vi "fit_data.vi"() -> ()   [LabVIEW 2013]
uses:
  <vilib>/Analysis/6fits.llb/Curve Fitting Criteria.ctl
  <vilib>/Analysis/6fits.llb/Confidence Interval (Linear).vi
  <vilib>/Utility/file.llb/Read From Spreadsheet File (DBL).vi
  <vilib>/Analysis/NI_AALPro.lvlib
panel:
  out "RMSE 2":dbl
  out "R-square":dbl
  out "SSE":dbl
  in  "confidence level":dbl=0.67 format="%.2f"
  out "delta intercept":dbl
  out "RMSE":dbl
  out "residue":dbl format="%#_3g"
  out "intercept":dbl
  out "XY Graph":T1(graph)
  in  "data file":path=path "C:/Users/Thermo/Documents/GitHub/HelixMC/MSControl/test_vis/fit_data_linear.txt"
  in  "Combo Box":string(combo)
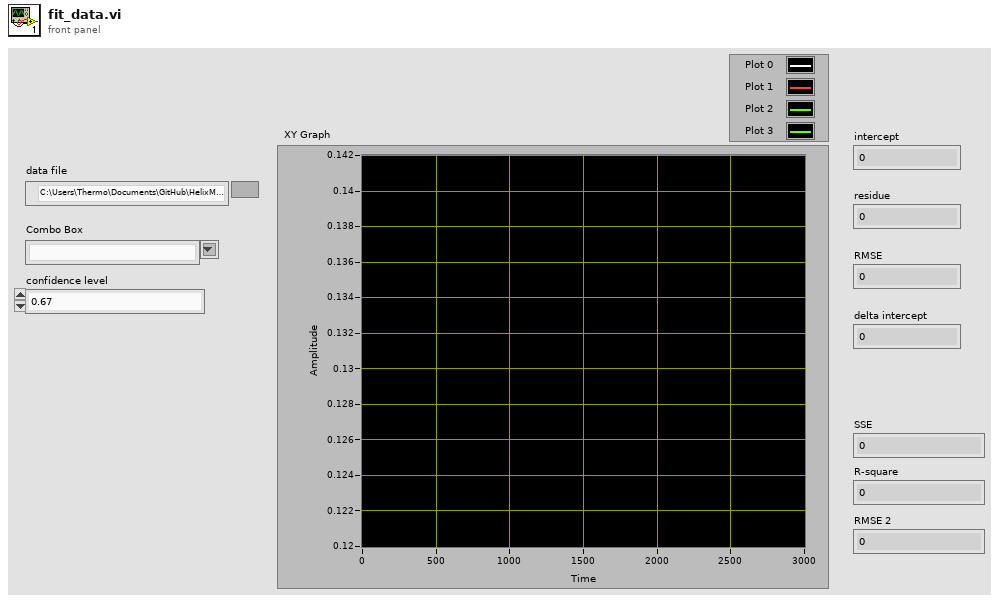
[diagram p1: front panel]
types:
  T1 = cluster{"all rows":dbl[], "Best Linear Fit":dbl[]}[]
  T2 = typedef "NI_AALPro.lvlib/Curve Fitting Criteria.ctl" = u16
  T3 = cluster{"all rows":dbl[], "Best Linear Fit":dbl[]}
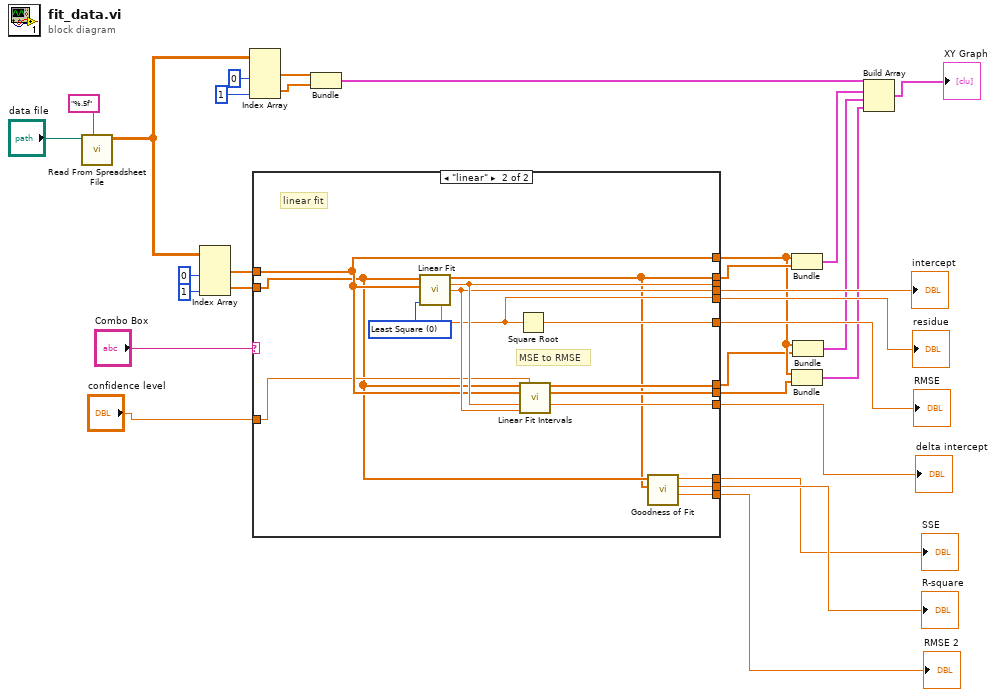
[diagram p0: block diagram]
diagram:
  n1 = call-poly <vilib>:"Read From Spreadsheet File.vi"("format (%.3f)"="%.5f", "file path (dialog if empty)"="data file") -> ("all rows"=w22:dbl[][])  [unwired: 5 in, 4 out]
  n2 = Index Array(array=w22, index (col) #1=0 ("disabled index (col)"), index (col) #2=1 ("index (col)")) -> (element #1=w24:dbl[], element #2=w23:dbl[])  [unwired: 2 in]
  n3 = Index Array(array=w22, index (col) #1=0 ("disabled index (col)"), index (col) #2=1 ("index (col)")) -> (element #1=w19:dbl[], element #2=w18:dbl[])  [unwired: 2 in]
  n4 = case shown="\"linear\"" "Combo Box" {
    tunnel: w24 -> [w30 w37]
    tunnel: w23 -> [_ w35]
    tunnel: [_ w34] -> w17
    tunnel: [_ w44] -> _
    tunnel: [_ w43] -> w13
    tunnel: [_ w42] -> w12
    tunnel: [_ w41] -> w11
    tunnel: [_ w40] -> w8
    tunnel: [_ w39] -> w7
    tunnel: [_ w38] -> w4
    tunnel: [w30 w37] -> w9
    tunnel: "confidence level" -> [_ w36]
    tunnel: [_ w33] -> w1
    tunnel: [_ w32] -> w3
    tunnel: [_ w31] -> w2
    frame "False", Default {
    }
    frame "linear" {
      w45 = T2 0 items=["Least Square", "Least Absolute Residual", "Bisquare"] ("method")
      # "MSE to RMSE"
      # "linear fit"
      n5 = call <vilib>:"Linear Fit.vi"("Y"=w35, "X"=w37, "method"=w45) -> ("Best Linear Fit"=w34:dbl[], "slope"=w44:dbl, "intercept"=w43:dbl, "residue"=w42:dbl)  [unwired: 8 in, 1 out]
      n6 = Square Root(x=w42) -> (sqrt(x)=w41:dbl)
      n7 = call-poly <vilib>:"Linear Fit Intervals.vi"("Y"=w35, "confidence level"=w36, "X"=w37, "slope"=w44, "intercept"=w43) -> ("Upper Bound"=w40:dbl[], "Lower Bound"=w39:dbl[], "delta intercept"=w38:dbl)  [unwired: 6 in, 2 out]
      n8 = call <vilib>:"Goodness of Fit.vi"("Best Fit"=w34, "Y"=w35) -> ("RMSE"=w31:dbl, "R-square"=w32:dbl, "SSE"=w33:dbl)  [unwired: 6 in, 1 out]
    }
  }
  "intercept" <- w13
  "residue" <- w12
  "RMSE" <- w11
  "delta intercept" <- w4
  "SSE" <- w1
  "R-square" <- w3
  "RMSE 2" <- w2
  n9 = Bundle("all rows"=w19, "all rows"=w18) -> (w16:cluster{"all rows":dbl[], "all rows":dbl[]})  [unwired: 1 in]
  n10 = Bundle("all rows"=w9, "Best Linear Fit"=w17) -> (w15:T3)  [unwired: 1 in]
  n11 = Bundle("all rows"=w9, "Lower Bound"=w7) -> (w5:cluster{"all rows":dbl[], "Lower Bound":dbl[]})  [unwired: 1 in]
  n12 = Bundle("all rows"=w9, "Upper Bound"=w8) -> (w6:cluster{"all rows":dbl[], "Upper Bound":dbl[]})  [unwired: 1 in]
  n13 = Build Array(w16, w15, w6, w5) -> (→"XY Graph":cluster{"all rows":dbl[], "Lower Bound":dbl[]}[])
